vi "Read.vi"(8 "Error In":errorcluster, 11 "VISA resource name":refnum<visa-resource-name>) -> (0 "Error Out":errorcluster, 2 "Read Data":string, 3 "VISA resource name out":refnum<visa-resource-name>)   [LabVIEW 2013]
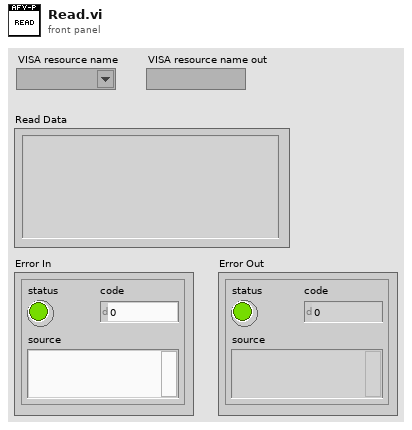
[diagram p1: front panel]
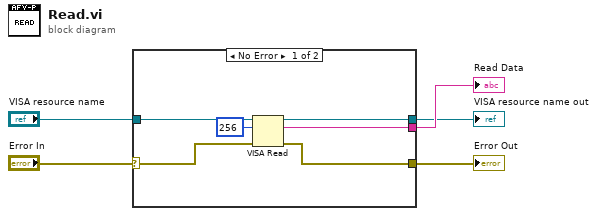
[diagram p0: block diagram]
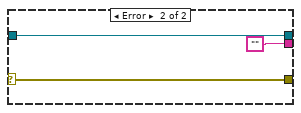
[diagram p2: hidden frame]
diagram:
  n1 = case shown="No Error" "Error In" {
    selector: "Error In" -> [w7 w14]
    tunnel: [w10 ""] -> w5
    tunnel: [w6 w14] -> w3
    tunnel: "VISA resource name" -> [w8 w12]
    tunnel: [w11 w12] -> w1
    frame No Error {
      n2 = VISA Read(VISA resource name=w8, byte count=u32 256, error in (no error)=w7) -> (VISA resource name out=w11:refnum<visa-resource-name>, read buffer=w10:string, error out=w6:errorcluster)  [unwired: 1 out]
    }
    frame Error {
    }
  }
  "Read Data" <- w5
  "Error Out" <- w3
  "VISA resource name out" <- w1
